vi "Actor Teardown.vi"(11 "Dev Actor in":refnum<class "Dev Actor.lvclass">) -> (2 "Teardown?":bool, 3 "Dev Actor out":refnum<class "Dev Actor.lvclass">)   [LabVIEW 2021, in "Dev Actor.lvlib" / "Dev Actor.lvclass"]
uses:
  Dev Actor.lvclass
  Dev Actor.lvclass/Dev Actor.ctl
  <vilib>/jettl/jettl/jettl/Actor/Actor.lvclass
  Panel/Panel.lvclass
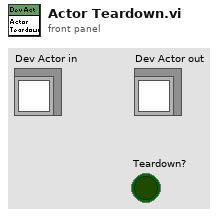
[diagram p1: front panel]
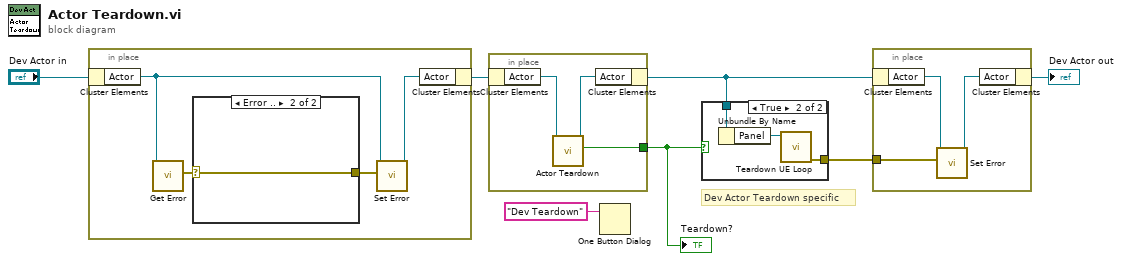
[diagram p0: block diagram]
diagram:
  # "Dev Actor Teardown specific"
  n1 = in-place {
    n2 = in-place-cluster #1("Dev Actor in") -> ("Actor"=w8:refnum<class "Actor.lvclass">)
    n3 = call-dynamic "Get Error.vi"("Actor in"=w8) -> ("Error"=w10:errorcluster)  [unwired: 10 in]
    n4 = case shown="Error .." w10 {
      selector: w10 -> [_ w12]
      tunnel: [_ w12] -> w9
      frame No Error {
      }
      frame Error {
      }
    }
    n5 = call-dynamic "Set Error.vi"("Error"=w9, "Actor in"=w8) -> ("Actor out"=w11:refnum<class "Actor.lvclass">)  [unwired: 9 in]
    n6 = in-place-cluster #1("Actor"=w11) -> (w1:refnum<class "Dev Actor.lvclass">)
  }
  n7 = in-place {
    in-place-border: [w13] -> w4
    n8 = in-place-cluster #2(w1) -> ("Actor"=w15:refnum<class "Actor.lvclass">)
    n9 = call-dynamic "Actor Teardown.vi"("Actor in"=w15) -> ("Teardown?"=w13:bool, "Actor out"=w14:refnum<class "Actor.lvclass">)  [unwired: 9 in]
    n10 = in-place-cluster #2("Actor"=w14) -> (w5:refnum<class "Dev Actor.lvclass">)
  }
  "Teardown?" <- w4
  n11 = One Button Dialog(message="Dev Teardown") -> ()  [unwired: 1 in, 1 out]
  n12 = case shown="True" w4 {
    tunnel: w5 -> [_ w18]
    tunnel: [_ w16] -> w3
    frame False {
    }
    frame True {
      n13 = Unbundle By Name(w18) -> ("Panel"=w17:refnum<class "Panel.lvclass">)
      n14 = call-dynamic "Teardown UE Loop.vi"("Panel in"=w17) -> ("error out"=w16:errorcluster)  [unwired: 10 in]
    }
  }
  n15 = in-place {
    in-place-border: w3 -> [w19]
    n16 = in-place-cluster #3(w5) -> ("Actor"=w21:refnum<class "Actor.lvclass">)
    n17 = call-dynamic "Set Error.vi"("Error"=w19, "Actor in"=w21) -> ("Actor out"=w20:refnum<class "Actor.lvclass">)  [unwired: 9 in]
    n18 = in-place-cluster #3("Actor"=w20) -> (→"Dev Actor out":refnum<class "Dev Actor.lvclass">)
  }
